vi "default error actions.vi"() -> (3 "default error responses":T1)   [LabVIEW 2013, in "Standard Engine Configuration.lvclass"]
uses:
  Standard Engine Configuration.lvclass
  Runtime/error responses.ctl
  error options.ctl
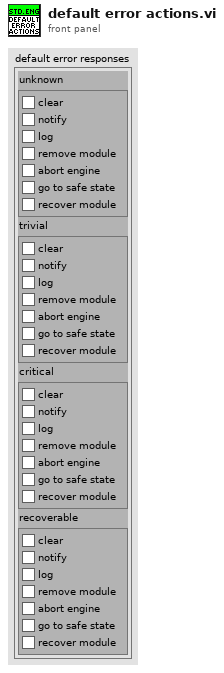
[diagram p1: front panel]
types:
  T1 = typedef "Standard Engine Configuration.lvclass/error responses.ctl" = cluster{"unknown":T2, "trivial":T2, "critical":T2, "recoverable":T2}
  T2 = typedef "Standard Engine Configuration.lvclass/error options.ctl" = cluster{"clear":bool, "notify":bool, "log":bool, "remove module":bool, "abort engine":bool, "go to safe state":bool, "recover module":bool}
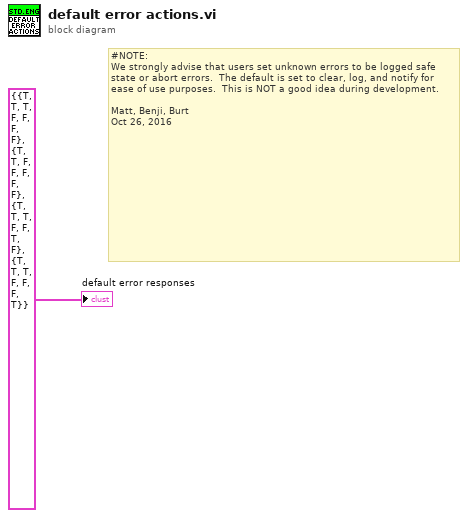
[diagram p0: block diagram]
diagram:
  # "#NOTE:\nWe strongly advise that users set unknown errors to be logged safe state or abort errors.  The default is set to clear, log, and notify for ease of use purposes.  This is NOT a good idea during development.\n\nMatt, Benji, Burt\nOct 26, 2016"
  "default error responses" <- T1 {"unknown"={"clear"=TRUE, "notify"=TRUE, "log"=TRUE, "remove module"=FALSE, "abort engine"=FALSE, "go to safe state"=FALSE, "recover module"=FALSE}, "trivial"={"clear"=TRUE, "notify"=TRUE, "log"=FALSE, "remove module"=FALSE, "abort engine"=FALSE, "go to safe state"=FALSE, "recover module"=FALSE}, "critical"={"clear"=TRUE, "notify"=TRUE, "log"=TRUE, "remove module"=FALSE, "abort engine"=FALSE, "go to safe state"=TRUE, "recover module"=FALSE}, "recoverable"={"clear"=TRUE, "notify"=TRUE, "log"=TRUE, "remove module"=FALSE, "abort engine"=FALSE, "go to safe state"=FALSE, "recover module"=TRUE}} ("default error responses")
